vi "ROIToolVisibility.vi"(3 "ROI Tool Button Visibility":T2) -> (0 "OK":bool, 1 "End ROI Tool Button Visibility":T1)   [LabVIEW 2009]
panel:
  in  "All Hidden":bool
  in  "All Visible":bool
  in  "Cancel":bool
  in  "OK":bool
  in  "ROI Tool Button Visibility Listbox":i32(listbox) caption="ROI Tool Button Visibility"
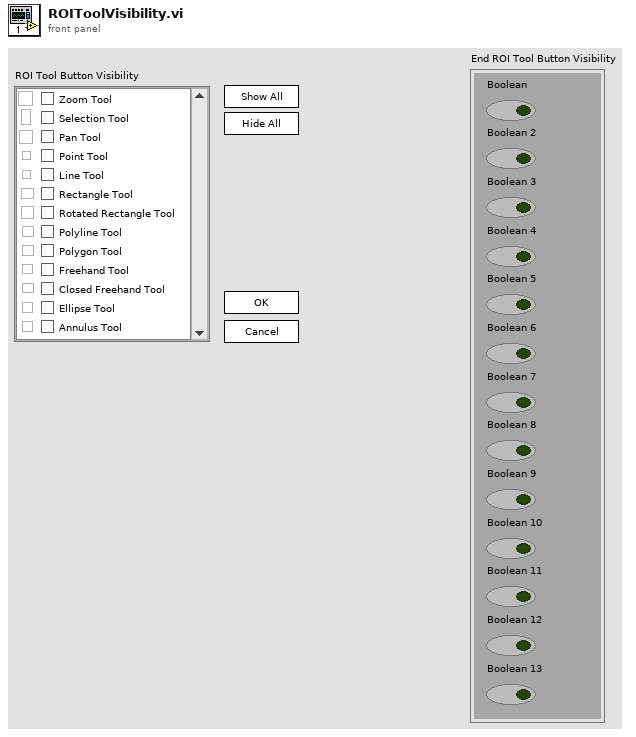
[diagram p1: front panel]
types:
  T1 = cluster{"Boolean":bool, "Boolean 2":bool, "Boolean 3":bool, "Boolean 4":bool, "Boolean 5":bool, "Boolean 6":bool, "Boolean 7":bool, "Boolean 8":bool, "Boolean 9":bool, "Boolean 10":bool, "Boolean 11":bool, "Boolean 12":bool, "Boolean 13":bool}
  T2 = cluster{"Zoom Tool":bool, "Selection Tool":bool, "Pan Tool":bool, "Point Tool":bool, "Line Tool":bool, "Rectangle Tool":bool, "Rotated Rectangle Tool":bool, "Polyline Tool":bool, "Polygon Tool":bool, "Freehand Tool":bool, "Closed Freehand Tool":bool, "Ellipse Tool":bool, "Annulus Tool":bool}
  T3 = enum32{"Invalid", "Standard", "Closed", "Hidden", "Minimized", "Maximized"}
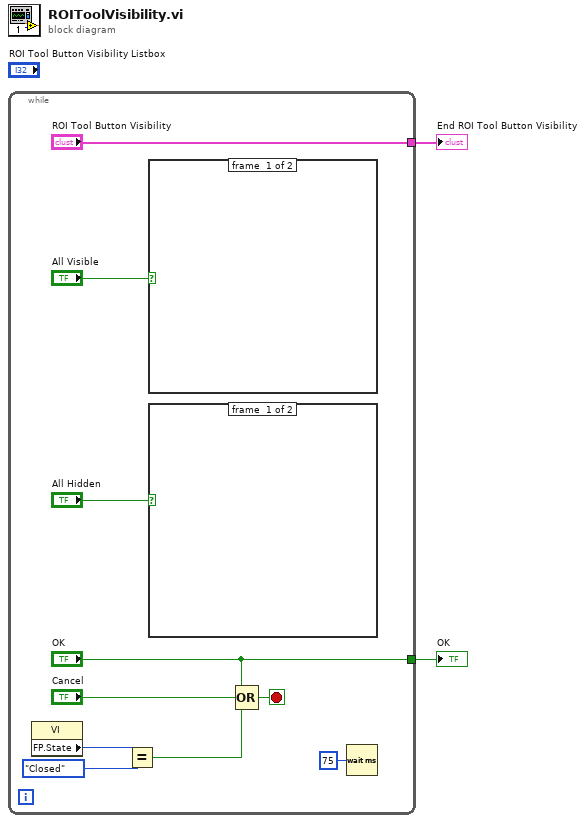
[diagram p0: block diagram]
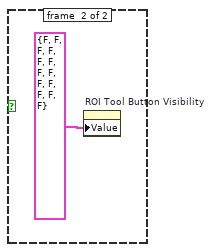
[diagram p2: hidden frame]
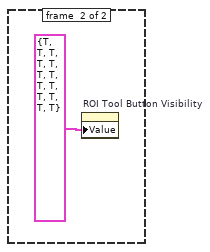
[diagram p3: hidden frame]
diagram:
  n1 = while {
    tunnel: ["OK"] -> w2
    tunnel: ["ROI Tool Button Visibility"] -> w1
    stop <- w12 stop-if-true
    n2 = property class="VI"() -> ("FP.State"=w5:T3)  [unwired: 2 in, 2 out]
    n3 = Equal?(x=w5, y=T3."Closed") -> (x = y?=w3:bool)
    n4 = case shown="True" "All Visible" {
      frame #0 {
      }
      frame #1 {
        n5 = property on="ROI Tool Button Visibility" class="Cluster (strict)"("Value"=T2 {"Zoom Tool"=TRUE, "Selection Tool"=TRUE, "Pan Tool"=TRUE, "Point Tool"=TRUE, "Line Tool"=TRUE, "Rectangle Tool"=TRUE, "Rotated Rectangle Tool"=TRUE, "Polyline Tool"=TRUE, "Polygon Tool"=TRUE, "Freehand Tool"=TRUE, "Closed Freehand Tool"=TRUE, "Ellipse Tool"=TRUE, "Annulus Tool"=TRUE} ("Value (Signaling)")) -> ()  [unwired: 2 in, 2 out]
      }
    }
    n6 = case shown="True" "All Hidden" {
      frame #0 {
      }
      frame #1 {
        n7 = property on="ROI Tool Button Visibility" class="Cluster (strict)"("Value"=T2 {"Zoom Tool"=FALSE, "Selection Tool"=FALSE, "Pan Tool"=FALSE, "Point Tool"=FALSE, "Line Tool"=FALSE, "Rectangle Tool"=FALSE, "Rotated Rectangle Tool"=FALSE, "Polyline Tool"=FALSE, "Polygon Tool"=FALSE, "Freehand Tool"=FALSE, "Closed Freehand Tool"=FALSE, "Ellipse Tool"=FALSE, "Annulus Tool"=FALSE} ("Value (Signaling)")) -> ()  [unwired: 2 in, 2 out]
      }
    }
    n8 = Compound Arithmetic op=OR("OK", "Cancel", w3) -> (w12:bool)
    n9 = Wait (ms)(milliseconds to wait=u32 75) -> ()  [unwired: 1 out]
  }
  "OK" <- w2
  "End ROI Tool Button Visibility" <- w1
